vi "Get Panel Ref.vi"(8 "error in (no error)":errorcluster, 11 "Panel In":refnum<class "Panel.lvclass">) -> (0 "error out":errorcluster, 2 "Panel Ref":refnum<vi>, 3 "Panel":refnum<class "Panel.lvclass">)   [LabVIEW 2018, in "OOPanel.lvlib" / "PanelManager.lvclass"]
uses:
  PanelManager.lvclass
  Panel/Panel.lvclass
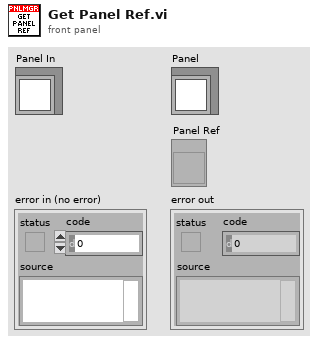
[diagram p1: front panel]
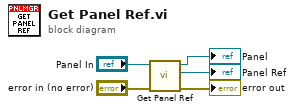
[diagram p0: block diagram]
diagram:
  n1 = call "Get Panel Ref.vi"("error in (no error)"="error in (no error)", "Panel in"="Panel In") -> ("error out"=→"error out":errorcluster, "Panel Ref"=→"Panel Ref":refnum<vi>, "Panel out"=→"Panel":refnum<class "Panel.lvclass">)  [unwired: 7 in]
